vi "FindCorners.vi"() -> ()   [LabVIEW 2018]
panel:
  out "Image to process":picture
  out "Processed image":picture
  out "Refined corners":cluster{"X":u32, "Y":dbl}[](array[cluster])
  out "Harris corners":cluster{"X":u32, "Y":dbl}[](array[cluster])
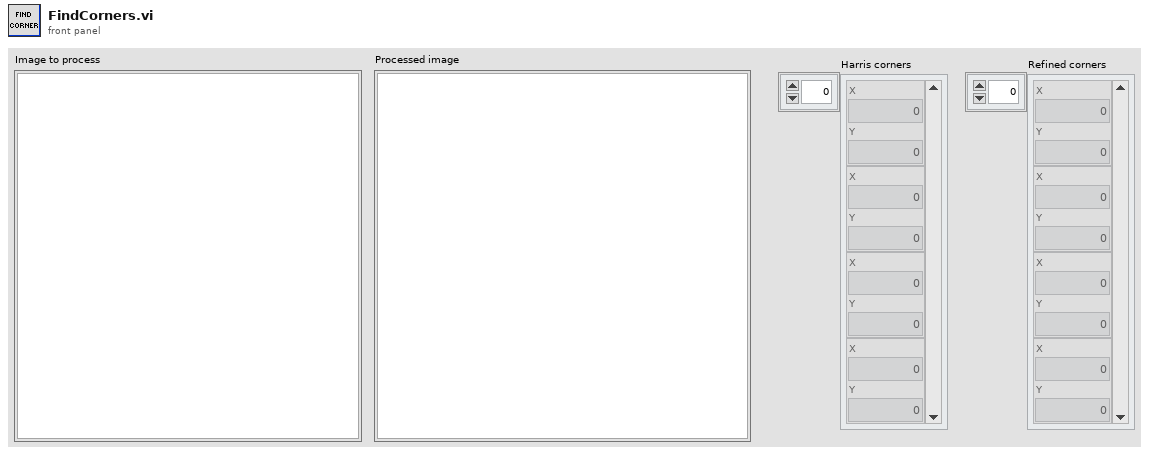
[diagram p1: front panel]
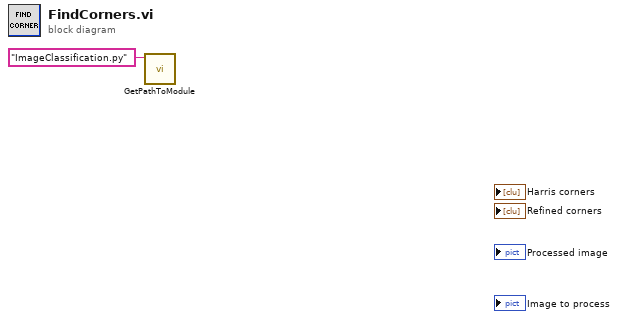
[diagram p0: block diagram]
diagram:
  n1 = call "GetPathToModule.vi"("module name"="ImageClassification.py") -> ()  [unwired: 10 in, 1 out]
